vi "绘制预览图片.vi"(8 "error in (no error)":errorcluster caption="错误输入（无错误）", 11 "程序 输入":refnum<class "程序.lvclass">) -> (0 "error out":errorcluster caption="错误输出", 3 "程序 输出":refnum<class "程序.lvclass">)   [LabVIEW 2018, in "程序.lvclass"]
uses:
  <vilib>/Utility/miscctls.llb/LVPoint32TypeDef.ctl
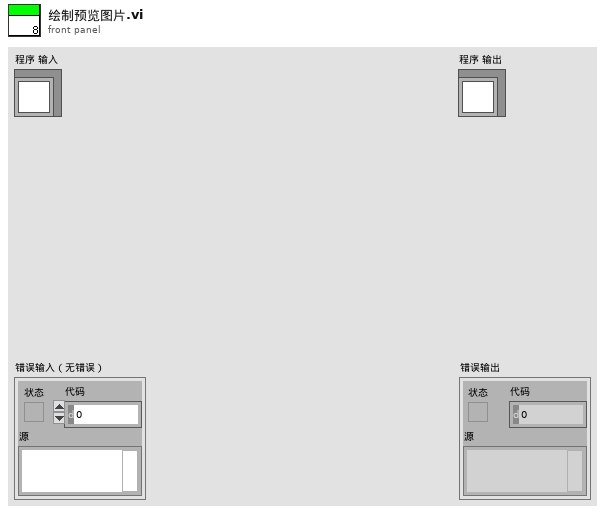
[diagram p1: front panel]
types:
  T1 = typedef "LVPoint32TypeDef.ctl" = cluster{"Horizontal":i32, "Vertical":i32}
  T2 = typedef "LVPositionTypeDef.ctl" = cluster{"Left":i32, "Top":i32}
  T3 = cluster{"图片":picture, "名称":string, "文本程序":string, "关键字":string}[][]
  T4 = typedef "LVBoundsTypeDef.ctl" = cluster{"Width":u32, "Height":u32}
  T5 = cluster{"图片":picture, "名称":string, "文本程序":string, "关键字":string}
  T6 = typedef "imagedata.ctl" = cluster{"image type":i32, "image depth":i32, "image":u8[], "mask":u8[], "colors":u32[], "Rectangle":cluster{"left":i16, "top":i16, "right":i16, "bottom":i16}}
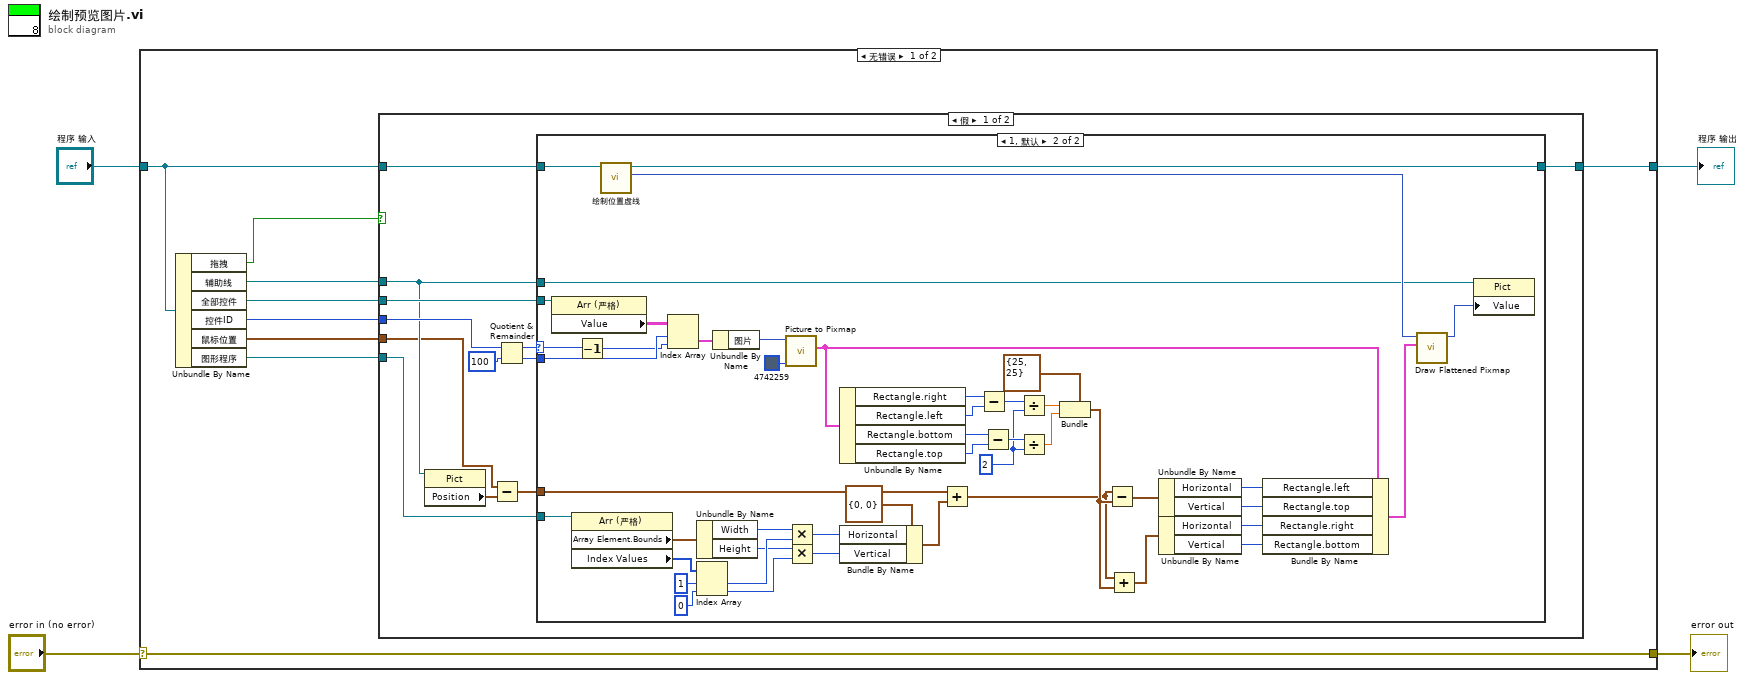
[diagram p0: block diagram]
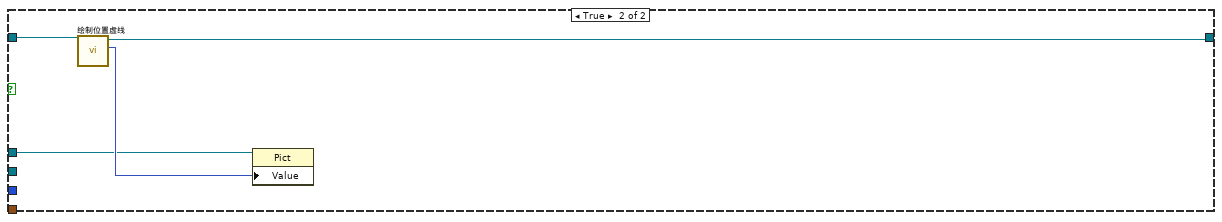
[diagram p3: hidden frame]
diagram:
  n1 = case shown="无错误" "error in (no error)" {
    selector: "error in (no error)" -> [w13 w79]
    tunnel: [w13 w79] -> w1
    tunnel: [w9 w78] -> w4
    tunnel: "程序 输入" -> [w10 w78]
    frame No Error {
      n2 = Unbundle By Name(w10) -> ("拖拽"=w5:bool, "辅助线"=w8:refnum<vi>, "全部控件"=w11:refnum<vi>, "控件ID"=w12:u32, "鼠标位置"=w7:T1, "图形程序"=w6:refnum<vi>)
      n3 = case shown="假" w5 {
        tunnel: w12 -> [w25 _]
        tunnel: w11 -> [w23 _]
        tunnel: w10 -> [w21 w77]
        tunnel: [w20 w76] -> w9
        tunnel: w8 -> [w19 w74]
        tunnel: w7 -> [w18 _]
        tunnel: w6 -> [w14 _]
        frame False {
          n4 = property class="Pict"(reference=w19) -> ("Position"=w17:T2)  [unwired: 1 in, 2 out]
          n5 = Subtract(x=w18, y=w17) -> (x-y=w16:T1)
          n6 = Quotient & Remainder(x=w25, y=u32 100) -> (x-y*floor(x/y)=w22:u32, floor(x/y)=w15:u32)
          n7 = case shown="1, 默认" w22 {
            selector: w22 -> [_ w70]
            tunnel: w19 -> [_ w56]
            tunnel: w23 -> [_ w71]
            tunnel: w16 -> [_ w28]
            tunnel: w21 -> [w26 w59]
            tunnel: [w26 w58] -> w20
            tunnel: w15 -> [_ w55]
            tunnel: w14 -> [_ w41]
            frame 0 {
            }
            frame 1, Default {
              w46 = i16 2 ("y")
              n8 = property class="Arr (严格)"(reference=w71) -> ("Value"=w73:T3)  [unwired: 1 in, 2 out]
              n9 = property class="Arr (严格)"(reference=w41) -> ("Array Element.Bounds"=w40:T4, "Index Values"=w39:u32[])  [unwired: 1 in, 2 out]
              n10 = Decrement(x=w70) -> (x-1=w54:u32)
              n11 = call-dynamic "绘制位置虚线.vi"("程序 输入"=w59) -> ("new picture"=w57:picture, "程序 输出"=w58:refnum<class "程序.lvclass">)  [unwired: 8 in, 1 out]
              n12 = Index Array(array=w73, index (row)=w55, index (col)=w54) -> (element=w72:T5)
              n13 = Unbundle By Name(w40) -> ("Width"=w36:u32, "Height"=w34:u32)
              n14 = Index Array(array=w39, index #1=1 ("索引"), index #2=0 ("索引")) -> (element #1=w35:u32, element #2=w33:u32)
              n15 = Unbundle By Name(w72) -> ("图片"=w62:picture)
              n16 = call <vilib>:"Picture to Pixmap.vi"("Background Color"=u32 4742259, "picture"=w62) -> ("image data"=w53:T6)  [unwired: 8 in, 1 out]
              n17 = Multiply(x=w36, y=w35) -> (x*y=w31:u32)
              n18 = Multiply(x=w34, y=w33) -> (x*y=w30:u32)
              n19 = Unbundle By Name(w53) -> ("Rectangle.right"=w52:i16, "Rectangle.left"=w51:i16, "Rectangle.bottom"=w50:i16, "Rectangle.top"=w49:i16)
              n20 = Bundle By Name(cluster=T1 {"Horizontal"=0, "Vertical"=0} ("鼠标位置"), "Horizontal"=w31, "Vertical"=w30) -> (w29:T1)
              n21 = Add(x=w28, y=w29) -> (x+y=w27:T1)
              n22 = Subtract(x=w52, y=w51) -> (x-y=w48:i16)
              n23 = Subtract(x=w50, y=w49) -> (x-y=w47:i16)
              n24 = Divide(x=w48, y=w46) -> (x/y=w45:dbl)
              n25 = Divide(x=w47, y=w46) -> (x/y=w44:dbl)
              n26 = Bundle(cluster=T1 {"Horizontal"=25, "Vertical"=25} ("y"), "Horizontal"=w45, "Vertical"=w44) -> (w42:T1)
              n27 = Subtract(x=w27, y=w42) -> (x-y=w69:T1)
              n28 = Add(x=w27, y=w42) -> (x+y=w68:T1)
              n29 = Unbundle By Name(w69) -> ("Horizontal"=w66:i32, "Vertical"=w65:i32)
              n30 = Unbundle By Name(w68) -> ("Horizontal"=w64:i32, "Vertical"=w63:i32)
              n31 = Bundle By Name(cluster=w53, "Rectangle.left"=w66, "Rectangle.top"=w65, "Rectangle.right"=w64, "Rectangle.bottom"=w63) -> (w67:T6)
              n32 = call <vilib>:"Draw Flattened Pixmap.vi"("image data"=w67, "picture"=w57) -> ("new picture"=w60:picture)  [unwired: 7 in]
              n33 = property class="Pict"(reference=w56, "Value"=w60) -> ()  [unwired: 1 in, 2 out]
            }
          }
        }
        frame True {
          n34 = call-dynamic "绘制位置虚线.vi"("程序 输入"=w77) -> ("new picture"=w75:picture, "程序 输出"=w76:refnum<class "程序.lvclass">)  [unwired: 8 in, 1 out]
          n35 = property class="Pict"(reference=w74, "Value"=w75) -> ()  [unwired: 1 in, 2 out]
        }
      }
    }
    frame Error {
    }
  }
  "error out" <- w1
  "程序 输出" <- w4
